vi "GetVoltage.vi"(8 "error in (no error)":errorcluster, 11 "TecellaChannel in":refnum<class "TecellaChannel.lvclass">) -> (0 "error out":errorcluster, 2 "Voltage (mV)":dbl, 3 "TecellaChannel out":refnum<class "TecellaChannel.lvclass">)   [LabVIEW 2009, in "TecellaChannel.lvclass"]
uses:
  TecellaChannel.lvclass
  TecellaChannel.lvclass/TecellaChannel.ctl
  TecellaClient/TecellaClient.lvclass
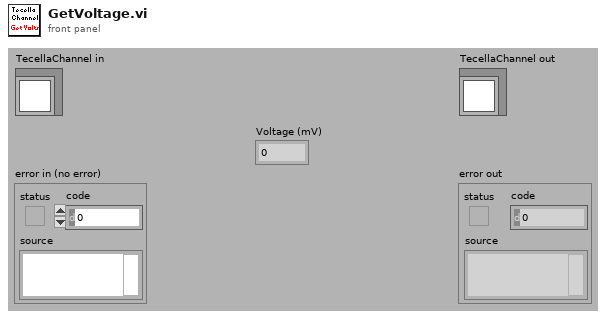
[diagram p1: front panel]
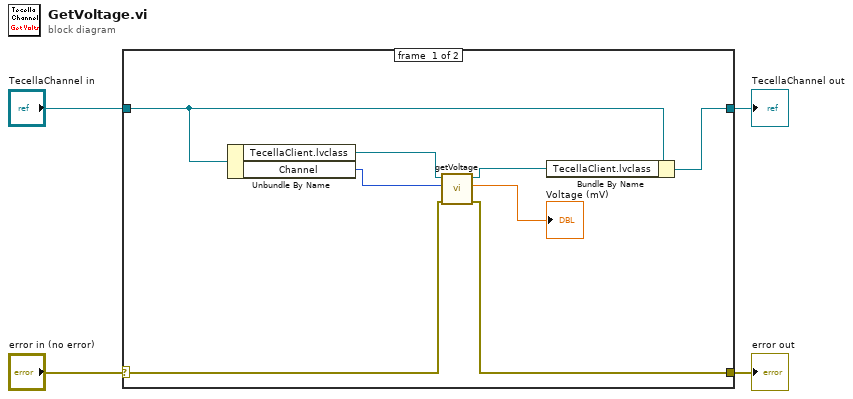
[diagram p0: block diagram]
diagram:
  n1 = case shown="No Error" "error in (no error)" {
    selector: "error in (no error)" -> [w6 w14]
    tunnel: [w5 w14] -> w3
    tunnel: [w11 w13] -> w1
    tunnel: "TecellaChannel in" -> [w12 w13]
    frame #0 {
      n2 = Unbundle By Name(w12) -> ("TecellaClient.lvclass"=w9:refnum<class "TecellaClient.lvclass">, "Channel"=w8:i8)
      n3 = call-dynamic "getVoltage.vi"("error in (no error)"=w6, "Channel"=w8, "TecellaClient in"=w9) -> ("error out"=w5:errorcluster, "Voltage (mV)"=→"Voltage (mV)":dbl, "TecellaClient out"=w10:refnum<class "TecellaClient.lvclass">)  [unwired: 6 in]
      n4 = Bundle By Name(cluster=w12, "TecellaClient.lvclass"=w10) -> (w11:refnum<class "TecellaChannel.lvclass">)
    }
    frame #1 {
    }
  }
  "error out" <- w3
  "TecellaChannel out" <- w1
